vi "ql2_query_to_id.vi"(11 "query_type":T1) -> (2 "query_type_ids":u32[](array[numeric]), 3 "id":u32)   [LabVIEW 2017, in "rethinkdb.lvlib"]
uses:
  rethinkdb.lvlib
  ql2_query.ctl
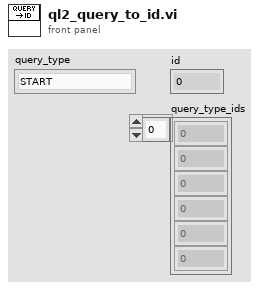
[diagram p1: front panel]
types:
  T1 = typedef "rethinkdb.lvlib/ql2_query.ctl" = enum8{"START", "CONTINUE", "STOP", "NOREPLY_WAIT", "SERVER_INFO", "invalid"}
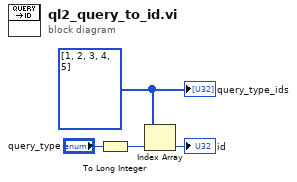
[diagram p0: block diagram]
diagram:
  w1 = u32[] [1, 2, 3, 4, 5] ("ids")
  n1 = To Long Integer(number="query_type") -> (32bit integer=w3:i32)
  n2 = Index Array(array=w1, index=w3) -> (element=→"id":u32)
  "query_type_ids" <- w1
